vi "generate transfer specifications.vi"(6 "paired tags":refnum<class "tag descriptor.lvclass">[](array[class]), 7 "main is source?":bool, 8 "error in":errorcluster, 9 "channels":refnum<class "TBM channel.lvclass">[](array[class]), 10 "dictionaries by class":refnum<class "data dictionary.lvclass">[](array[class]), 11 "main data dictionary":refnum<class "data dictionary.lvclass">) -> (0 "error out":errorcluster, 3 "transfer specifications":cluster{"transfer specification":T1[]}[](array[cluster]))   [LabVIEW 2013, in "Standard Engine Runtime.lvclass"]
doc: "Performs the lookups required to generate a transfer spec for one set of channels."
uses:
  Standard Engine Runtime.lvclass
  <vilib>/NI/Tag Bus/table/transfer specification.ctl
  <vilib>/NI/Tag Bus/tag/Data Type.ctl
  <vilib>/NI/Tag Bus/dictionary/data dictionary.lvclass
  <vilib>/NI/Tag Bus Module Framework/channel/TBM channel.lvclass
  <vilib>/NI/Tag Bus/tag/tag descriptor.lvclass
  <vilib>/NI/Tag Bus/tag/tag descriptor.lvclass/tag descriptor.ctl
  <vilib>/NI/Tag Bus/tag/read tag name.vi
  <vilib>/NI/Tag Bus/dictionary/locate tag.vi
  <vilib>/NI/Tag Bus/table/data table.lvlib
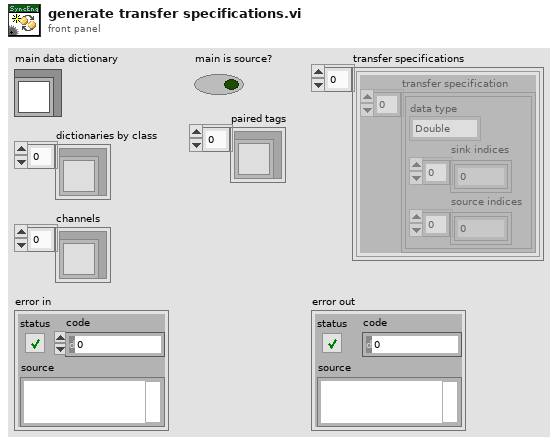
[diagram p1: front panel]
types:
  T1 = typedef "tag bus.lvlib/data table.lvlib/transfer specification.ctl" = cluster{"data type":T2, "sink indices":i32[], "source indices":i32[]}
  T2 = typedef "tag bus.lvlib/tag descriptor.lvclass/Data Type.ctl" = enum16{"Double", "Single", "I64", "I32", "I16", "I8", "U64", "U32", "U16", "U8", "Boolean", "String", "Array of Double", "Array of Single", "Array of I64", "Array of I32", "Array of I16", "Array of I8", "Array of U64", "Array of U32", "Array of U16", "Array of U8", "Array of Boolean", "Array of String"}
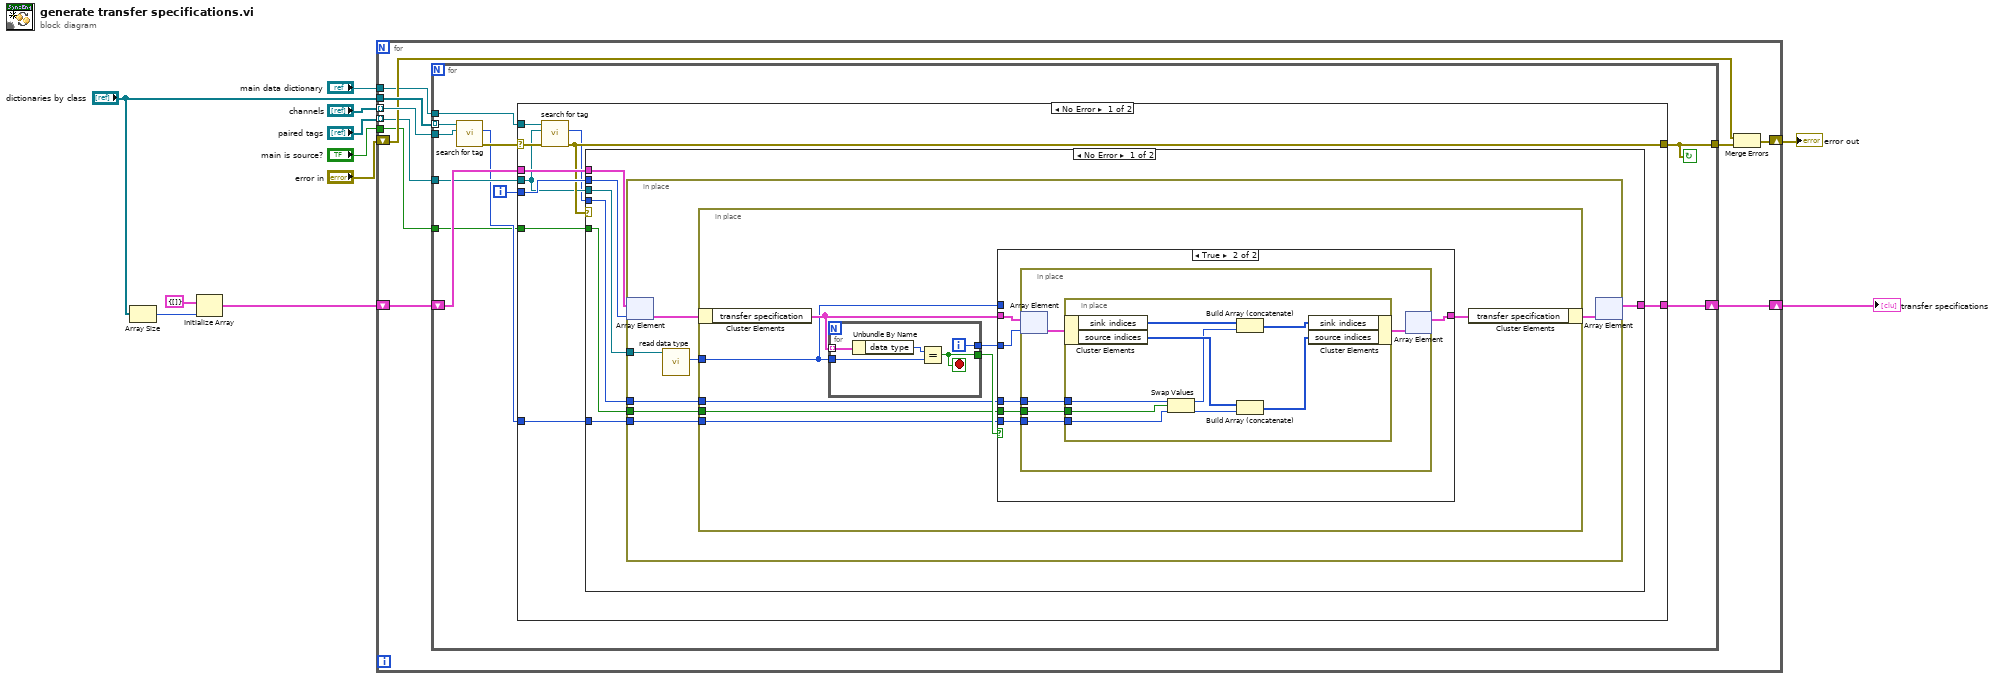
[diagram p0: block diagram]
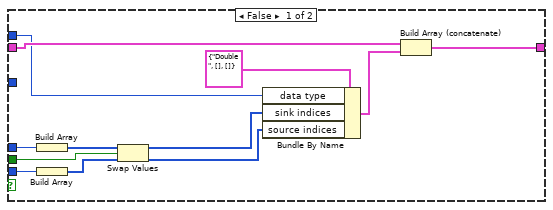
[diagram p2: hidden frame]
diagram:
  n1 = Array Size(array="dictionaries by class") -> (size(s)=w7:i32)
  n2 = Initialize Array(cluster{"transfer specification":T1[]} {"transfer specification"=[]}, w7) -> (w5:cluster{"transfer specification":T1[]}[])
  n3 = for {
    tunnel: "channels" -> [w19] mode=indexing
    tunnel: "dictionaries by class" -> [w21]
    shift-right: [w16] -> w4
    shift-left: w5 -> [w20]
    shift-right: [w18] -> w11
    shift-left: "error in" -> [w17]
    tunnel: "paired tags" -> [w13] mode=indexing
    tunnel: "main data dictionary" -> [w14]
    tunnel: "main is source?" -> [w12]
    n4 = for {
      tunnel: w21 -> [w32] mode=indexing
      shift-right: [w27] -> w16
      shift-left: w20 -> [w29]
      tunnel: w19 -> [w31]
      tunnel: [w28] -> w15
      tunnel: w14 -> [w25]
      tunnel: w13 -> [w24]
      tunnel: w12 -> [w22]
      i -> [w26]
      stop <- w28 continue-if-true
      n5 = call <vilib>:"search for tag.vi"("system tag"=w31, "data dictionary in"=w32) -> ("error out"=w30:errorcluster, "index"=w23:i32)  [unwired: 7 in, 1 out]
      n6 = case shown="No Error" w30 {
        selector: w30 -> [w39 w104]
        tunnel: w29 -> [w42 w103]
        tunnel: [w37 w104] -> w28
        tunnel: [w41 w103] -> w27
        tunnel: w26 -> [w40 _]
        tunnel: w25 -> [w38 _]
        tunnel: w24 -> [w36 _]
        tunnel: w23 -> [w34 _]
        tunnel: w22 -> [w33 _]
        frame No Error {
          n7 = call <vilib>:"search for tag.vi"("error in"=w39, "system tag"=w36, "data dictionary in"=w38) -> ("error out"=w37:errorcluster, "index"=w35:i32)  [unwired: 6 in, 1 out]
          n8 = case shown="No Error" w37 {
            tunnel: w42 -> [w49 w102]
            tunnel: [w48 w102] -> w41
            tunnel: w40 -> [w47 _]
            tunnel: w36 -> [w46 _]
            tunnel: w35 -> [w45 _]
            tunnel: w34 -> [w44 _]
            tunnel: w33 -> [w43 _]
            frame No Error {
              n9 = in-place {
                in-place-border: w46 -> [w56]
                in-place-border: w45 -> [w52]
                in-place-border: w44 -> [w51]
                in-place-border: w43 -> [w50]
                n10 = in-place-array #1(w49, w47) -> (w55:cluster{"transfer specification":T1[]})
                n11 = call <vilib>:"read data type.vi"("system tag in"=w56) -> ("data type"=w53:T2)  [unwired: 8 in, 2 out]
                n12 = in-place {
                  in-place-border: w53 -> [w61]
                  in-place-border: w52 -> [w60]
                  in-place-border: w51 -> [w59]
                  in-place-border: w50 -> [w58]
                  n13 = in-place-cluster #2(w55) -> ("transfer specification"=w63:T1[])
                  n14 = for {
                    tunnel: w63 -> [w101] mode=indexing
                    tunnel: w61 -> [w100]
                    tunnel: [w98] -> w57
                    tunnel: [w97] -> w64
                    i -> [w98]
                    stop <- w97 stop-if-true
                    n15 = Unbundle By Name(w101) -> ("data type"=w99:T2)
                    n16 = Equal?(x=w99, y=w100) -> (x = y?=w97:bool)
                  }
                  n17 = case shown="True" w64 {
                    tunnel: w63 -> [w76 w82]
                    tunnel: [w75 w80] -> w62
                    tunnel: w61 -> [w72 _]
                    tunnel: w60 -> [w71 w78]
                    tunnel: w59 -> [w70 w77]
                    tunnel: w58 -> [w65 w79]
                    tunnel: w57 -> [_ w81]
                    frame False {
                      n18 = Build Array(w71) -> (w69:i32[])
                      n19 = Build Array(w70) -> (w68:i32[])
                      n20 = Swap Values(12:w69, 13:w65, 14:w68) -> (1:w67:i32[], 3:w66:i32[])
                      n21 = Bundle By Name(cluster=T1 {"data type"=enum."Double", "sink indices"=[], "source indices"=[]} ("merge specification"), "data type"=w72, "sink indices"=w67, "source indices"=w66) -> (w73:T1)
                      n22 = Build Array (concatenate)(w76, w73) -> (w75:T1[])
                    }
                    frame True {
                      n23 = in-place {
                        in-place-border: w79 -> [w85]
                        in-place-border: w78 -> [w84]
                        in-place-border: w77 -> [w83]
                        n24 = in-place-array #3(w82, w81) -> (w87:T1)
                        n25 = in-place {
                          in-place-border: w85 -> [w96]
                          in-place-border: w84 -> [w95]
                          in-place-border: w83 -> [w94]
                          n26 = in-place-cluster #4(w87) -> ("sink indices"=w90:i32[], "source indices"=w93:i32[])
                          n27 = Swap Values(12:w95, 13:w96, 14:w94) -> (1:w89:i32, 3:w88:i32)
                          n28 = Build Array (concatenate)(w90, w89) -> (w91:i32[])
                          n29 = Build Array (concatenate)(w93, w88) -> (w92:i32[])
                          n30 = in-place-cluster #4("sink indices"=w91, "source indices"=w92) -> (w86:T1)
                        }
                        n31 = in-place-array #3(w86) -> (w80:T1[])  [unwired: 1 out]
                      }
                    }
                  }
                  n32 = in-place-cluster #2("transfer specification"=w62) -> (w54:cluster{"transfer specification":T1[]})
                }
                n33 = in-place-array #1(w54) -> (w48:cluster{"transfer specification":T1[]}[])  [unwired: 1 out]
              }
            }
            frame Error {
            }
          }
        }
        frame Error {
        }
      }
    }
    n34 = Merge Errors(w17, w15) -> (w18:errorcluster)
  }
  "error out" <- w11
  "transfer specifications" <- w4
